vi "SmartInsert QuickDrop.vi"(6 "Variant in":variant, 7 "Shift Pressed?":bool, 8 "error in (no error)":errorcluster, 10 "QD Combo Box Ref":refnum<vi>, 11 "QD Launch VI Ref":refnum<vi>) -> (0 "error out":errorcluster, 4 "Variant out":variant)   [LabVIEW 2014]
doc: "This quickdrop functionality will insert the selected node in the selected wire. Make sure that selected wire and node terminals have same data type.\n\nDefault Shortcut - [1]"
panel:
  in  "Undo Name":string="Quick Drop Keyboard Shortcut"
  # "Do not change the connector pane of this VI.\n\nSee the block diagram for directions on how to use this template."
  # "Specify the name of the Undo transaction"
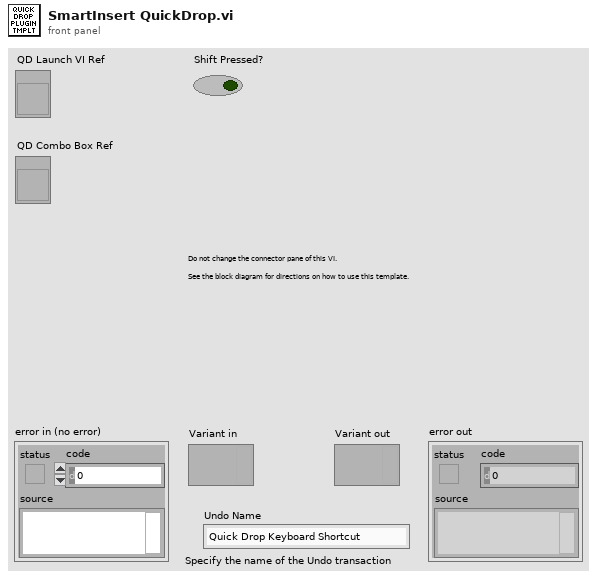
[diagram p1: front panel]
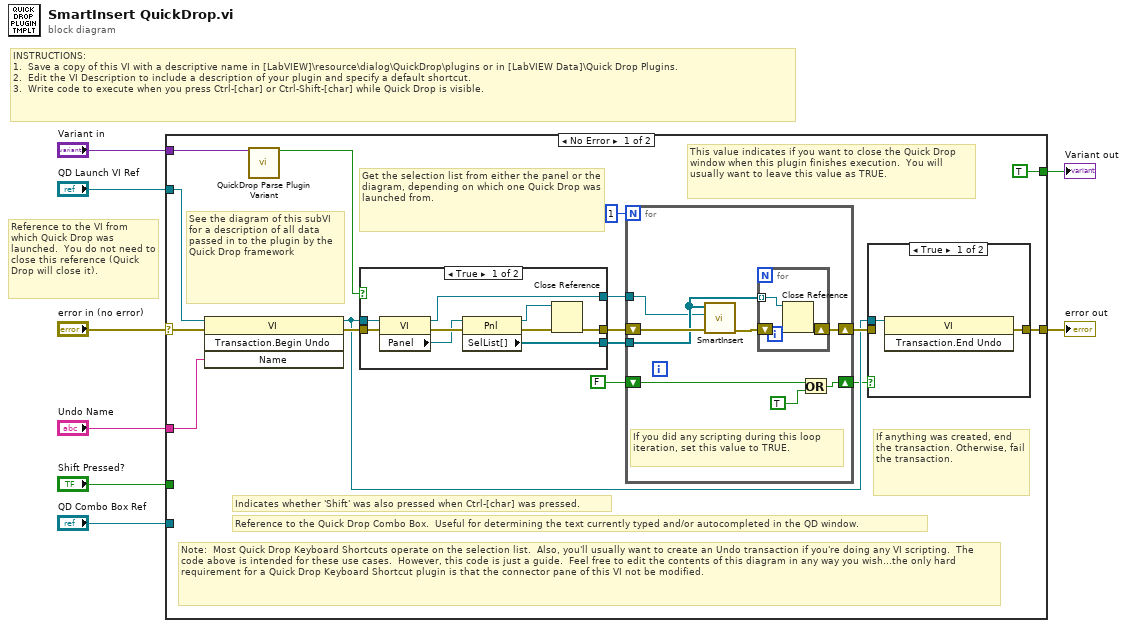
[diagram p0: block diagram]
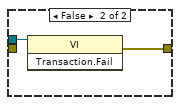
[diagram p2: hidden frame]
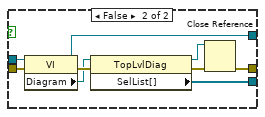
[diagram p3: hidden frame]
diagram:
  # "Reference to the VI from which Quick Drop was launched.  You do not need to close this reference (Quick Drop will close it)."
  # "INSTRUCTIONS:\n1.  Save a copy of this VI with a descriptive name in [LabVIEW]\\resource\\dialog\\QuickDrop\\plugins or in [LabVIEW Data]\\Quick Drop Plugins.\n2.  Edit the VI Description to include a description of your plugin and specify a default shortcut. \n3.  Write code to execute when you press Ctrl-[char] or Ctrl-Shift-[char] while Quick Drop is visible."
  n1 = case shown="No Error" "error in (no error)" {
    selector: "error in (no error)" -> [w23 w58]
    tunnel: [w17 w58] -> w7
    tunnel: "QD Launch VI Ref" -> [w22 _]
    tunnel: "Shift Pressed?" -> [_ _]
    tunnel: "QD Combo Box Ref" -> [_ _]
    tunnel: "Variant in" -> [w24 _]
    tunnel: "Undo Name" -> [w21 _]
    tunnel: [TRUE _] -> w1
    frame No Error {
      # "Note:  Most Quick Drop Keyboard Shortcuts operate on the selection list.  Also, you'll usually want to create an Undo transaction if you're doing any VI scripting.  The code above is intended for these use cases.  However, this code is just a guide.  Feel free to edit the contents of this diagram in any way you wish...the only hard requirement for a Quick Drop Keyboard Shortcut plugin is that the connector pane of this VI not be modified."
      # "Get the selection list from either the panel or the diagram, depending on which one Quick Drop was launched from."
      # "If anything was created, end the transaction. Otherwise, fail the transaction."
      # "This value indicates if you want to close the Quick Drop window when this plugin finishes execution.  You will usually want to leave this value as TRUE."
      # "See the diagram of this subVI for a description of all data passed in to the plugin by the Quick Drop framework"
      # "Reference to the Quick Drop Combo Box.  Useful for determining the text currently typed and/or autocompleted in the QD window."
      # "Indicates whether 'Shift' was also pressed when Ctrl-[char] was pressed."
      n2 = invoke on="Invoke Node" class="VI" method="Transaction.Begin Undo"(reference=w22, error in=w23, "Name"=w21) -> (reference out=w14:refnum<vi>, error out=w18:errorcluster)  [unwired: 1 in, 2 out]
      n3 = call <vilib>:"QuickDrop Parse Plugin Variant.vi"("QDKS Variant in"=w24) -> ("QD Launch VI Panel?"=w19:bool)  [unwired: 12 in, 2 out]
      n4 = case shown="True" w19 {
        tunnel: w18 -> [w48 w57]
        tunnel: w14 -> [w47 w56]
        tunnel: [w42 w51] -> w16
        tunnel: [w41 w50] -> w11
        tunnel: [w40 w49] -> w9
        frame True {
          n5 = property on="Property Node" class="VI"(reference=w47, error in=w48) -> (reference out=w40:refnum<vi>, error out=w46:errorcluster, "Panel"=w45:refnum<vi>)
          n6 = property on="Property Node" class="Pnl"(reference=w45, error in=w46) -> (reference out=w43:refnum<vi>, error out=w44:errorcluster, "SelList[]"=w41:refnum<vi>[])
          n7 = Close Reference(reference=w43, error in (no error)=w44) -> (error out=w42:errorcluster)
        }
        frame False {
          n8 = property on="Property Node" class="VI"(reference=w56, error in=w57) -> (reference out=w49:refnum<vi>, error out=w55:errorcluster, "Diagram"=w54:refnum<vi>)
          n9 = property on="Property Node" class="TopLvlDiag"(reference=w54, error in=w55) -> (reference out=w52:refnum<vi>, error out=w53:errorcluster, "SelList[]"=w50:refnum<vi>[])
          n10 = Close Reference(reference=w52, error in (no error)=w53) -> (error out=w51:errorcluster)
        }
      }
      n11 = for {
        N: 1 -> [_]
        shift-right: [w29] -> w15
        shift-left: w16 -> [w28]
        shift-right: [w31] -> w12
        shift-left: FALSE -> [w32]
        tunnel: w11 -> [w26]
        tunnel: w9 -> [w25]
        # "If you did any scripting during this loop iteration, set this value to TRUE."
        n12 = call "SmartInsert.vi"("error in (no error)"=w28, "VI reference In"=w25, "SelList[]"=w26) -> ("error out"=w27:errorcluster)  [unwired: 8 in]
        n13 = for {
          shift-right: [w35] -> w29
          shift-left: w27 -> [w34]
          tunnel: w26 -> [w33] mode=indexing
          n14 = Close Reference(reference=w33, error in (no error)=w34) -> (error out=w35:errorcluster)
        }
        n15 = Or(x=w32, y=TRUE ("x")) -> (x .or. y?=w31:bool)
      }
      n16 = case shown="True" w12 {
        tunnel: w14 -> [w36 w38]
        tunnel: [w37 w39] -> w17
        tunnel: w15 -> [_ _]
        frame True {
          n17 = invoke on="Invoke Node" class="VI" method="Transaction.End Undo"(reference=w36) -> (error out=w37:errorcluster)  [unwired: 2 in, 2 out]
        }
        frame False {
          n18 = invoke on="Invoke Node" class="VI" method="Transaction.Fail"(reference=w38) -> (error out=w39:errorcluster)  [unwired: 2 in, 2 out]
        }
      }
    }
    frame Error {
    }
  }
  "error out" <- w7
  "Variant out" <- w1
